vi "ShowHidePicCtrl.vi"(8 "图例类型":enum16{"图例", "游标", "统计", "峰值"}(ring), 10 "状态":bool, 11 "PicCtrlRef":refnum<vi>) -> ()   [LabVIEW 2012, in "WaveGraphX.xctl"]
uses:
  WaveGraphX.xctl
  <vilib>/Utility/miscctls.llb/LVPositionTypeDef.ctl
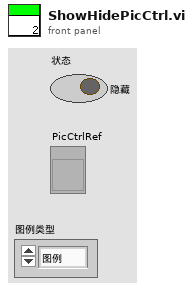
[diagram p1: front panel]
types:
  T1 = typedef "LVPositionTypeDef.ctl" = cluster{"Left":i32, "Top":i32}
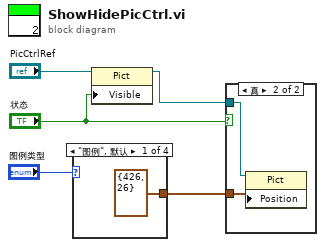
[diagram p0: block diagram]
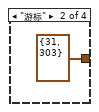
[diagram p2: hidden frame]
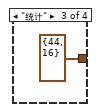
[diagram p3: hidden frame]
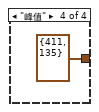
[diagram p4: hidden frame]
diagram:
  n1 = case shown="\"图例\", 默认" "图例类型" {
    tunnel: [T1 {"Left"=426, "Top"=26} ("位置") T1 {"Left"=31, "Top"=303} ("位置") T1 {"Left"=44, "Top"=16} ("位置") T1 {"Left"=411, "Top"=135} ("位置")] -> w1
    frame "图例", Default {
    }
    frame "游标" {
    }
    frame "统计" {
    }
    frame "峰值" {
    }
  }
  n2 = property class="Pict"(reference="PicCtrlRef", "Visible"="状态") -> (reference out=w3:refnum<vi>)  [unwired: 1 in, 1 out]
  n3 = case shown="真" "状态" {
    tunnel: w3 -> [_ w11]
    tunnel: w1 -> [_ w10]
    frame False {
    }
    frame True {
      n4 = property class="Pict"(reference=w11, "Position"=w10) -> ()  [unwired: 1 in, 2 out]
    }
  }
